vi "LAS-CTS_2dScan.vi"() -> ()   [LabVIEW 2024]
doc: "Shows how to move a motor to an absolute position."
uses:
  C:/Users/Behna/OneDrive/Documents/LAS/LAS-Labview-Controls/LAS LV Scan/Kinesis/Thorlabs.MotionControl.Controls.dll
  Kinesis/Thorlabs.MotionControl.Controls.dll
  <vilib>/Analysis/baseanly.llb/Mean (DBL).vi
  C:/Users/Behna/OneDrive/Documents/LAS/LAS-Labview-Controls/LAS LV Scan/Kinesis/ThorLabs.MotionControl.KCube.DCServoCLI.dll
  Kinesis/ThorLabs.MotionControl.KCube.DCServoCLI.dll
  <vilib>/httpClient/LabVIEWHTTPClient.lvlib
  <vilib>/Analysis/NI_AALBase.lvlib
panel:
  out "Filename":path
  in  "File #":i32 format="%03d"
  in  "base filename":string
  in  "Filepath":path
  in  "Target ID":string
  out "Laser Energy (uJ)":dbl format="%#.3f"
  out "Pulses Remaining":i32
  out "Laser On/Off":bool
  in  "Energy Meter VISA port":refnum<visa-resource-name>="IntegraEnergyMeter"
  in  "KCubeDCServoControl Z axis":refnum<k24>(container)
  in  "KCubeDCServoControl X axis":refnum<k24>(container)
  out "Time Remaining (min)":dbl format="%#_2f"
  out "sec per spot":dbl
  out "scan started":bool
  out "Scan Progress":u8(slide) scale=0.0..42.0
  out "Scan Time (hr)":dbl format="%#_2f"
  in  "Number of Laser Pulses":i32=100
  in  "X Start Position":dbl=5.0
  in  "Z Start Position":dbl=4.0
  in  "Z Step Size (um)":dbl=500.0
  in  "# of Z Positions":i32=2
  in  "# of X Positions":i32=2
  in  "X Step Size (um)":dbl=500.0
  out "CurrentPosZ":dbl=6.0
  out "CurrentPosX":dbl=6.0
  in  "SerialNumber Z":string="27261646"
  in  "SerialNumber X":string="27261828"
  # "Connection Setup"
  # "Scan Parameters"
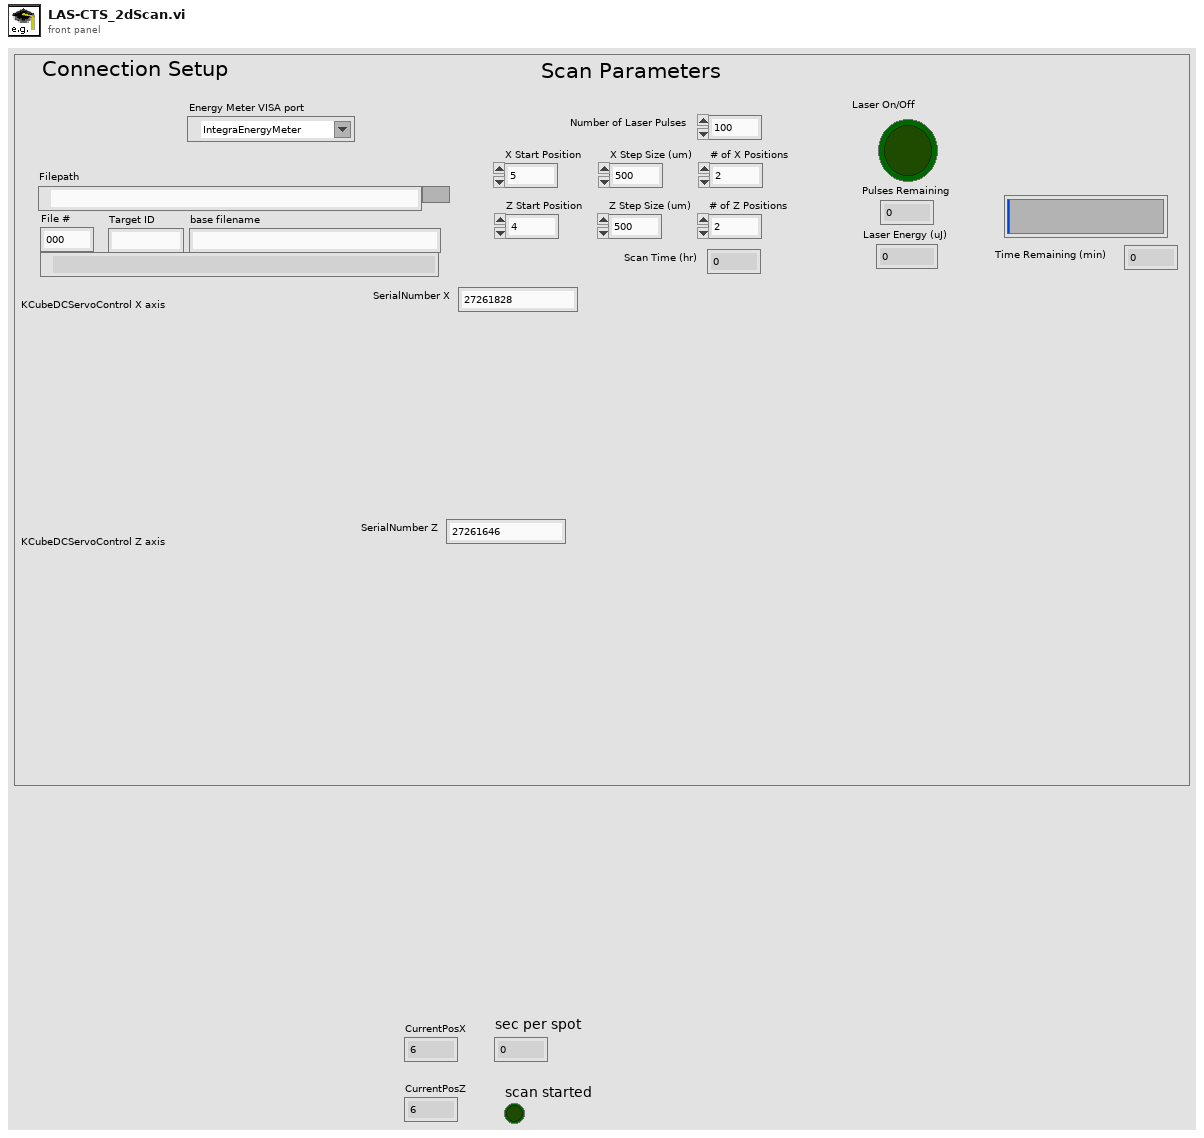
[diagram p1: front panel]
types:
  T1 = enum16{"open", "replace", "create", "open or create", "replace or create", "replace or create with confirmation"}
  T2 = typedef "LabVIEWHTTPClient.lvlib/ClientHandle.ctl" = refnum<k1>
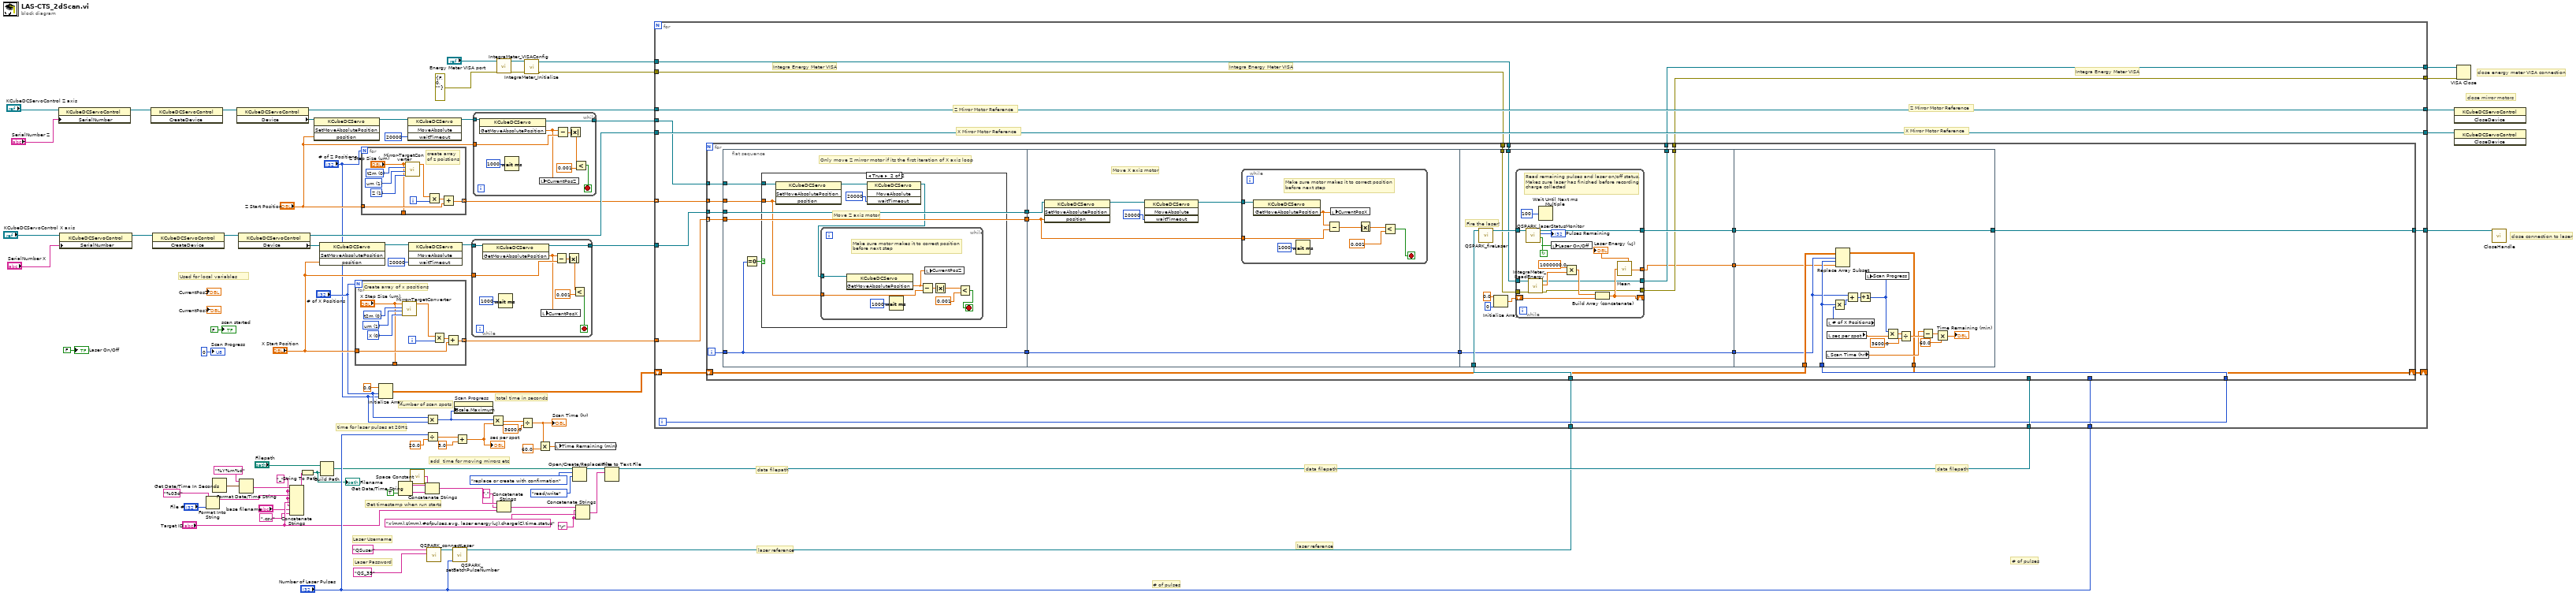
[diagram p0: block diagram]
diagram:
  w9 = "_" ("string")
  w27 = "\r"
  # "Get timestamp when run starts"
  # "close energy meter VISA connection"
  # "total time in seconds"
  # "add  time for moving mirrors etc"
  # "number of scan spots"
  # "time for laser pulses at 20Hz"
  # "data filepath"
  # "data filepath"
  # "close mirror motors"
  # "close connection to laser"
  # "Used for local variables"
  # "data filepath"
  # "laser reference"
  # "# of pulses"
  # "# of pulses"
  # "laser reference"
  # "Laser Password"
  # "Laser Username"
  n1 = property class="KCubeDCServoControl"(reference="KCubeDCServoControl Z axis", "SerialNumber"="SerialNumber Z") -> (reference out=w82:refnum<k24>)  [unwired: 1 in, 1 out]
  n2 = property class="KCubeDCServoControl"(reference="KCubeDCServoControl X axis", "SerialNumber"="SerialNumber X") -> (reference out=w85:refnum<k24>)  [unwired: 1 in, 1 out]
  n3 = invoke class="KCubeDCServoControl" method="CreateDevice"(reference=w82) -> (reference out=w76:refnum<k24>)  [unwired: 2 in, 2 out]
  n4 = invoke class="KCubeDCServoControl" method="CreateDevice"(reference=w85) -> (reference out=w83:refnum<k24>)  [unwired: 2 in, 2 out]
  n5 = Format Into String(format string="%03d", "File #") -> (resulting string=w12:string)  [unwired: 2 in, 1 out]
  n6 = Get Date/Time In Seconds() -> (seconds since 1Jan1904=w17:timestamp)
  n7 = property class="KCubeDCServoControl"(reference=w76) -> (reference out=w73:refnum<k24>, "Device"=w4:refnum<k24>)  [unwired: 1 in, 1 out]
  n8 = property class="KCubeDCServoControl"(reference=w83) -> (reference out=w72:refnum<k24>, "Device"=w65:refnum<k24>)  [unwired: 1 in, 1 out]
  n9 = Format Date/Time String(time format string (%c)="%Y%m%d", seconds (now)=w17) -> (date/time string=w15:string)  [unwired: 1 in]
  n10 = Concatenate Strings(w15, w9, w12, w9, "Target ID", w9, "base filename", ".csv" ("string")) -> (w18:string)
  n11 = String To Path(string=w18) -> (path=w6:path)
  "Filename" <- w6
  n12 = invoke class="KCubeDCServo" method="SetMoveAbsolutePosition"(reference=w4, "position"="Z Start Position") -> (reference out=w69:refnum<k24>)  [unwired: 2 in, 3 out]
  n13 = invoke class="KCubeDCServo" method="SetMoveAbsolutePosition"(reference=w65, "position"="X Start Position") -> (reference out=w67:refnum<k24>)  [unwired: 2 in, 3 out]
  n14 = Build Path(base path="Filepath", name or relative path=w6) -> (appended path=w11:path)
  n15 = for {
    N: "# of X Positions" -> [_]
    tunnel: [w90] -> w45 mode=indexing
    tunnel: "X Start Position" -> [w87]
    tunnel: ["X Step Size (um)"] -> _
    i -> [w88]
    w94 = u16 0 items=["X", "Z"] ("axis")
    w92 = u16 0 items=["t2m", "m2t"] ("Conversion")
    w93 = u16 1 items=["mm", "um"] ("input units")
    # "Create array of x positions"
    n16 = call "Mirror-TargetConverter.vi"("axis"=w94, "input units"=w93, "Conversion"=w92, "input distance"="X Step Size (um)") -> ("output distance"=w89:dbl)  [unwired: 7 in]
    n17 = Multiply(x=w89, y=w88) -> (x*y=w91:dbl)
    n18 = Add(x=w91, y=w87) -> (x+y=w90:dbl)
  }
  n19 = for {
    N: "# of Z Positions" -> [_]
    tunnel: [w97] -> w46 mode=indexing
    tunnel: "Z Start Position" -> [w96]
    tunnel: ["Z Step Size (um)"] -> _
    i -> [w103]
    w101 = u16 1 items=["X", "Z"] ("axis")
    w100 = u16 0 items=["t2m", "m2t"] ("Conversion")
    w102 = u16 1 items=["mm", "um"] ("input units")
    # "create array\nof z poistions"
    n20 = call "Mirror-TargetConverter.vi"("axis"=w101, "input units"=w102, "Conversion"=w100, "input distance"="Z Step Size (um)") -> ("output distance"=w99:dbl)  [unwired: 7 in]
    n21 = Multiply(x=w99, y=w103) -> (x*y=w98:dbl)
    n22 = Add(x=w98, y=w96) -> (x+y=w97:dbl)
  }
  n23 = Initialize Array(0.0, "# of X Positions", "# of Z Positions") -> (w36:dbl[][])
  n24 = Get Date/Time String(want seconds? (F)=TRUE) -> (date string=w26:string, time string=w25:string)  [unwired: 2 in]
  n25 = invoke class="KCubeDCServo" method="MoveAbsolute"(reference=w69, "waitTimeout"=20000) -> (reference out=w61:refnum<k24>)  [unwired: 2 in, 3 out]
  n26 = invoke class="KCubeDCServo" method="MoveAbsolute"(reference=w67, "waitTimeout"=20000) -> (reference out=w64:refnum<k24>)  [unwired: 2 in, 3 out]
  n27 = call <vilib>:"Space Constant.vi"() -> ("String"=w24:string)
  n28 = Multiply(x="# of X Positions", y="# of Z Positions") -> (x*y=w44:i32)
  n29 = Divide(x="Number of Laser Pulses", y=20.0) -> (x/y=w51:dbl)
  n30 = Concatenate Strings(w26, w24, w25) -> (w22:string)
  n31 = call "QSPARK_connectLaser.vi"("password"="QS_35", "username"="QSuser") -> ("client handle out"=w3:T2)  [unwired: 9 in]
  n32 = call "QSPARK_setBatchPulseNumber.vi"("Number of Pulses"="Number of Laser Pulses", "client handle"=w3) -> ("client handle out"=w59:T2)  [unwired: 9 in]
  n33 = property on="Scan Progress" class="Slide (strict)"("Scale.Maximum"=w44) -> ()  [unwired: 2 in, 2 out]
  n34 = Add(x=w51, y=3.0) -> (x+y=w49:dbl)
  "sec per spot" <- w49
  n35 = while {
    tunnel: w64 -> [w112]
    tunnel: "X Start Position" -> [w110]
    tunnel: [w109] -> w62
    stop <- w106 stop-if-true
    n36 = invoke class="KCubeDCServo" method="GetMoveAbsolutePosition"(reference=w112) -> (reference out=w109:refnum<k24>, "GetMoveAbsolutePosition"=w104:dbl)  [unwired: 2 in, 1 out]
    n37 = Wait (ms)(milliseconds to wait=u32 1000) -> ()  [unwired: 1 out]
    n38 = local write "CurrentPosX"(w104) -> ()
    n39 = Subtract(x=w104, y=w110) -> (x-y=w105:dbl)
    n40 = Absolute Value(x=w105) -> (abs(x)=w108:dbl)
    n41 = Less?(x=w108, y=0.001) -> (x < y?=w106:bool)
  }
  n42 = while {
    tunnel: w61 -> [w121]
    tunnel: "Z Start Position" -> [w117]
    tunnel: [w114] -> w60
    stop <- w119 stop-if-true
    n43 = invoke class="KCubeDCServo" method="GetMoveAbsolutePosition"(reference=w121) -> (reference out=w114:refnum<k24>, "GetMoveAbsolutePosition"=w116:dbl)  [unwired: 2 in, 1 out]
    n44 = Wait (ms)(milliseconds to wait=u32 1000) -> ()  [unwired: 1 out]
    n45 = local write "CurrentPosZ"(w116) -> ()
    n46 = Subtract(x=w116, y=w117) -> (x-y=w113:dbl)
    n47 = Absolute Value(x=w113) -> (abs(x)=w120:dbl)
    n48 = Less?(x=w120, y=0.001) -> (x < y?=w119:bool)
  }
  n49 = Multiply(x=w44, y=w49) -> (x*y=w48:dbl)
  n50 = call "IntegraMeter_VISAConfig.vi"("error in (no error)"=errorcluster {"status"=FALSE, "code"=0, "source"=""}, "VISA resource name"="Energy Meter VISA port") -> ("error out"=w33:errorcluster, "reference out"=w32:refnum<visa-resource-name>)  [unwired: 8 in]
  n51 = Concatenate Strings(w22, "," ("string"), "Target ID") -> (w20:string)
  n52 = Divide(x=w48, y=3600.0) -> (x/y=w40:dbl)
  "Scan Time (hr)" <- w40
  n53 = call "IntegraMeter_Initialize.vi"("error in"=w33, "VISA resource name"=w32) -> ("error out"=w30:errorcluster, "VISA resource name out"=w31:refnum<visa-resource-name>)  [unwired: 8 in]
  n54 = Multiply(x=w40, y=60.0) -> (x*y=w41:dbl)
  n55 = local write "Time Remaining (min)"(w41) -> ()
  n56 = Open/Create/Replace File(file path (use dialog)=w11, operation (0:open)=T1."replace or create with confirmation", access (0:read/write)=enum16{"read/write", "read-only", "write-only"}."read/write") -> (refnum out=w78:refnum<file>)  [unwired: 3 in, 2 out]
  n57 = Concatenate Strings(w20, w27, "x(mm),z(mm),#ofpulses,avg. laser energy(uJ),charge(C),time,status", w27) -> (w70:string)
  n58 = Write to Text File(file (use dialog)=w78, text=w70) -> (refnum out=w77:refnum<file>)  [unwired: 2 in, 2 out]
  n59 = for {
    tunnel: w62 -> [w138]
    tunnel: w46 -> [w130] mode=indexing
    tunnel: [w137] -> w81
    tunnel: w77 -> [w136]
    tunnel: "Number of Laser Pulses" -> [w135]
    tunnel: w45 -> [w134]
    tunnel: [w133] -> w75
    tunnel: [w132] -> w74
    tunnel: w73 -> [w133]
    tunnel: w72 -> [w132]
    tunnel: w60 -> [w129]
    tunnel: w59 -> [w131]
    shift-right: [w126] -> _
    shift-left: w36 -> [w127]
    tunnel: w31 -> [w125]
    tunnel: w30 -> [w124]
    tunnel: [w123] -> w29
    tunnel: [w122] -> w28
    i -> [w128]
    # "Integra Energy Meter VISA"
    # "Integra Energy Meter VISA"
    # "Integra Energy Meter VISA"
    # "X Mirror Motor Reference"
    # "X Mirror Motor Reference"
    # "Z Mirror Motor Reference"
    # "Z Mirror Motor Reference"
    n60 = for {
      tunnel: w138 -> [w159]
      tunnel: w134 -> [w158] mode=indexing
      tunnel: [w157] -> w137
      tunnel: w136 -> [_]
      tunnel: w135 -> [_]
      tunnel: w131 -> [w156]
      tunnel: w130 -> [w153]
      tunnel: w129 -> [w152]
      tunnel: w128 -> [w149]
      shift-right: [w147] -> w126
      shift-left: w127 -> [w148]
      tunnel: w125 -> [w146]
      tunnel: w124 -> [w145]
      tunnel: [w144] -> w123
      tunnel: [w143] -> w122
      i -> [w151]
      n61 = flat-sequence {
        tunnel: w158 -> [w161]
        tunnel: w159 -> [w162]
        tunnel: [w162] -> w155
        tunnel: [w161] -> w154
        tunnel: w153 -> [w165]
        tunnel: w152 -> [w164]
        tunnel: w151 -> [w160]
        tunnel: [w160] -> w150
        tunnel: w154 -> [w183]
        tunnel: w155 -> [w182]
        tunnel: [w179] -> w142
        tunnel: w150 -> [w179]
        tunnel: [w204] -> w141
        tunnel: w156 -> [w203]
        tunnel: [w201] -> w140
        tunnel: w142 -> [w201]
        tunnel: w146 -> [w197]
        tunnel: w145 -> [w196]
        tunnel: [w195] -> w144
        tunnel: [w194] -> w143
        tunnel: [w193] -> w139
        tunnel: [w237] -> w157
        tunnel: w141 -> [w237]
        tunnel: w140 -> [w233]
        tunnel: w149 -> [w235]
        tunnel: w148 -> [w236]
        tunnel: [w225] -> w147
        tunnel: w139 -> [w220]
        frame #0 {
          # "Only move Z mirror motor if its the first iteration of X axis loop"
          n62 = Equal To 0?(x=w160) -> (x = 0?=w163:bool)
          n63 = case shown="True" w163 {
            tunnel: w165 -> [_ w168]
            tunnel: w164 -> [_ w167]
            frame False {
            }
            frame True {
              # "Move Z axis motor"
              n64 = invoke class="KCubeDCServo" method="SetMoveAbsolutePosition"(reference=w167, "position"=w168) -> (reference out=w170:refnum<k24>)  [unwired: 2 in, 3 out]
              n65 = invoke class="KCubeDCServo" method="MoveAbsolute"(reference=w170, "waitTimeout"=20000) -> (reference out=w166:refnum<k24>)  [unwired: 2 in, 3 out]
              n66 = while {
                tunnel: w168 -> [w175]
                tunnel: w166 -> [w171]
                stop <- w176 stop-if-true
                # "Make sure motor makes it to correct position\nbefore next step"
                n67 = invoke class="KCubeDCServo" method="GetMoveAbsolutePosition"(reference=w171) -> ("GetMoveAbsolutePosition"=w172:dbl)  [unwired: 2 in, 2 out]
                n68 = Wait (ms)(milliseconds to wait=u32 1000) -> ()  [unwired: 1 out]
                n69 = Subtract(x=w172, y=w175) -> (x-y=w173:dbl)
                n70 = local write "CurrentPosZ"(w172) -> ()
                n71 = Absolute Value(x=w173) -> (abs(x)=w177:dbl)
                n72 = Less?(x=w177, y=0.001) -> (x < y?=w176:bool)
              }
            }
          }
        }
        frame #1 {
          # "Move X axis motor"
          n73 = invoke class="KCubeDCServo" method="SetMoveAbsolutePosition"(reference=w182, "position"=w183) -> (reference out=w181:refnum<k24>)  [unwired: 2 in, 3 out]
          n74 = invoke class="KCubeDCServo" method="MoveAbsolute"(reference=w181, "waitTimeout"=20000) -> (reference out=w184:refnum<k24>)  [unwired: 2 in, 3 out]
          n75 = while {
            tunnel: w184 -> [w191]
            tunnel: w183 -> [w189]
            stop <- w187 stop-if-true
            # "Make sure motor makes it to correct position\nbefore next step"
            n76 = invoke class="KCubeDCServo" method="GetMoveAbsolutePosition"(reference=w191) -> ("GetMoveAbsolutePosition"=w185:dbl)  [unwired: 2 in, 2 out]
            n77 = Wait (ms)(milliseconds to wait=u32 1000) -> ()  [unwired: 1 out]
            n78 = Subtract(x=w185, y=w189) -> (x-y=w190:dbl)
            n79 = local write "CurrentPosX"(w185) -> ()
            n80 = Absolute Value(x=w190) -> (abs(x)=w188:dbl)
            n81 = Less?(x=w188, y=0.001) -> (x < y?=w187:bool)
          }
        }
        frame #2 {
          # "Fire the laser!"
          n82 = call "QSPARK_fireLaser.vi"("client handle"=w203) -> ("client handle out"=w202:T2)  [unwired: 10 in]
          n83 = Initialize Array(0.0 ("element"), 0 ("dimension size")) -> (w198:dbl[])
          n84 = while {
            tunnel: w202 -> [w218]
            tunnel: [w217] -> w204
            shift-right: [w211] -> _
            shift-left: w198 -> [w214]
            tunnel: [w209] -> w193
            tunnel: w197 -> [w208]
            tunnel: w196 -> [w207]
            tunnel: [w206] -> w195
            tunnel: [w205] -> w194
            stop <- w215 continue-if-true
            # "Read remaining pulses and laser on/off status. \nMakes sure laser has finished before recording \ncharge collected"
            n85 = call "QSPARK_laserStatusMonitor.vi"("client handle"=w218) -> ("laser on?"=w215:bool, "remaining pulses"=→"Pulses Remaining":i32, "client handle out"=w217:T2)  [unwired: 8 in]
            n86 = call "IntegraMeter_ReadEnergy.vi"("error in (no error)"=w207, "VISA resource name"=w208) -> ("error out"=w205:errorcluster, "Laser Energy (J)"=w212:dbl, "VISA resource name out"=w206:refnum<visa-resource-name>)  [unwired: 7 in]
            n87 = Wait Until Next ms Multiple(millisecond multiple=u32 100) -> ()  [unwired: 1 out]
            n88 = local write "Laser On/Off"(w215) -> ()
            n89 = Multiply(x=1000000.0, y=w212) -> (x*y=w210:dbl)
            n90 = Build Array (concatenate)(w210, w214) -> (w211:dbl[])
            n91 = call-poly <vilib>:"Mean.vi"("X"=w211) -> ("mean"=w209:dbl)  [unwired: 1 out]
            "Laser Energy (uJ)" <- w209
          }
        }
        frame #3 {
          n92 = local read "Scan Time (hr)"() -> (w226:dbl)
          n93 = local read "# of X Positions"() -> (w231:i32)
          n94 = local read "sec per spot"() -> (w230:dbl)
          n95 = Multiply(x=w235, y=w231) -> (x*y=w234:i32)
          n96 = Replace Array Subset(array=w236, new element=w220, index (row)=w233, index (col)=w235) -> (w225:dbl[][])
          n97 = Add(x=w233, y=w234) -> (x+y=w232:i32)
          n98 = Increment(x=w232) -> (x+1=w224:i32)
          n99 = local write "Scan Progress"(w224) -> ()
          n100 = Multiply(x=w224, y=w230) -> (x*y=w229:dbl)
          n101 = Divide(x=w229, y=3600.0) -> (x/y=w227:dbl)
          n102 = Subtract(x=w226, y=w227) -> (x-y=w223:dbl)
          n103 = Multiply(x=w223, y=60.0) -> (x*y=→"Time Remaining (min)":dbl)
        }
      }
    }
  }
  n104 = invoke class="KCubeDCServoControl" method="CloseDevice"(reference=w75) -> ()  [unwired: 2 in, 3 out]
  n105 = invoke class="KCubeDCServoControl" method="CloseDevice"(reference=w74) -> ()  [unwired: 2 in, 3 out]
  n106 = VISA Close(VISA resource name=w29, error in (no error)=w28) -> ()  [unwired: 1 out]
  n107 = call <vilib>:"CloseHandle.vi"("client handle"=w81) -> ()  [unwired: 14 in, 1 out]
  "Laser On/Off" <- FALSE ("Laser On/Off")
  "scan started" <- FALSE
  "Scan Progress" <- u8 0 ("Scan Progress")
